vi "Convert Test Paramter Cluster to Listbox Contents.vi"(10 "Experiment Parameter Values (default)":T1(array[cluster])) -> (1 "2D String Array":string[][](array[string]), 2 "Parameter Names":string[](array[string]))   [LabVIEW 2014, in "Core SubVIs.lvlib"]
uses:
  Core SubVIs.lvlib
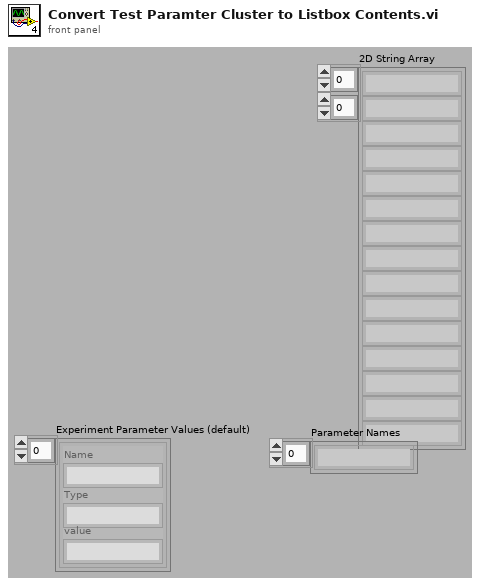
[diagram p1: front panel]
types:
  T1 = cluster{"Name":string, "Type":string, "value":string}[]
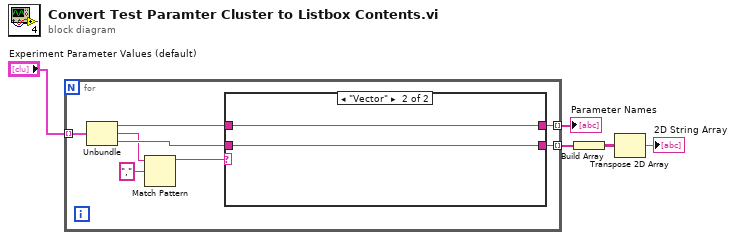
[diagram p0: block diagram]
diagram:
  n1 = for {
    tunnel: [w13] -> w4 mode=indexing
    tunnel: "Experiment Parameter Values (default)" -> [w12] mode=indexing
    tunnel: [w10] -> w1 mode=indexing
    n2 = Unbundle(w12) -> ("Name"=w11:string, "Type"=w6:string, "value"=w9:string)
    n3 = Match Pattern(string=w6, regular expression=",") -> (before substring=w7:string)  [unwired: 4 out]
    n4 = case shown="\"Vector\"" w7 {
      tunnel: [w14 w17] -> w13
      tunnel: w9 -> [w14 w17]
      tunnel: w11 -> [w15 w16]
      tunnel: [w15 w16] -> w10
      frame "String", Default {
      }
      frame "Vector" {
      }
    }
  }
  "Parameter Names" <- w1
  n5 = Build Array(w4) -> (w5:string[][])
  n6 = Transpose 2D Array(2D array=w5) -> (transposed array=→"2D String Array":string[][])
